vi "Teleop - Gyro Tracking (SubVI).vi"(0 "turretAngleDesiredInput":dbl=229.0, 1 "hoodAngleDesired In":dbl, 2 "shooterVelocityDesired In":dbl, 3 "shootNow In":bool, 4 "Constant Cluster In":T1 {"32. shooterHoodAngleRange" format="%_6f"; "31. turretAngleRange" format="%_6f"; "30. shooterVelocityLowerLimit" format="%_6f"; "29. shooterVelocityUpperLimit" format="%_6f"; "28. Robot Track Width (inches)" format="%_6f"; "27. Shooter Spin Up Speed (RPM)" format="%_6f"; "26. Climb Down Speed %" format="%_6f"; "25. Climb Up Speed %" format="%_6f"; "24. wallShooterVelocity" format="%_6f"; "23. Intake Spit Speed %" format="%_6f"; "22. Intake Suck Speed %" format="%_6f"; "21. CP Wheel Diameter" format="%_6f"; "20. Clockwise CP Fudge" format="%_6f"; "19. CouterClockwise CP Fudge" format="%_6f"; "18. Inches per Sector" format="%_6f"; "17. Ticks/Rotation Neo 550" format="%_6f"; "16. Control Panel Wheel Diameter" format="%_6f"; "15. Center-Center Sector Distance" format="%_6f"; "14. Inches / Tick Drivetrain" format="%_6f"; "13. Auton I Output Limit Drive Straight Gain" format="%_6f"; "12. Auton Deriv Drive Straight Gain" format="%_6f"; "11. Auton Int Drive Straight Gain" format="%_6f"; "10. Auton Prop Drive Straight Gain" format="%_6f"; "9. Auton I Output Limit Turn Gain" format="%_6f"; "8. Auton Deriv Turn Gain" format="%_6f"; "7. Auton Int Turn Gain" format="%_6f"; "1. Auton Prop Drive Gain" format="%_6f"; "2. Auton Int Drive Gain" format="%_6f"; "3. Auton Deriv Drive Gain" format="%_6f"; "4. I Output Drive  Limit" format="%_6f"; "5. Auto Drive Cheat (%)" format="%_6f"; "6. Auton Prop Turn Gain" format="%_6f"}, 5 "sensors In":T2) -> (15 "hoodAngleDesired Out":dbl, 16 "turretAngleDesiredOutput":dbl, 17 "shootNow Output":bool, 18 "Constant Cluster Out":T1 {"32. shooterHoodAngleRange" format="%_6f"; "31. turretAngleRange" format="%_6f"; "30. shooterVelocityLowerLimit" format="%_6f"; "29. shooterVelocityUpperLimit" format="%_6f"; "28. Robot Track Width (inches)" format="%_6f"; "27. Shooter Spin Up Speed (RPM)" format="%_6f"; "26. Climb Down Speed %" format="%_6f"; "25. Climb Up Speed %" format="%_6f"; "24. wallShooterVelocity" format="%_6f"; "23. Intake Spit Speed %" format="%_6f"; "22. Intake Suck Speed %" format="%_6f"; "21. CP Wheel Diameter" format="%_6f"; "20. Clockwise CP Fudge" format="%_6f"; "19. CouterClockwise CP Fudge" format="%_6f"; "18. Inches per Sector" format="%_6f"; "17. Ticks/Rotation Neo 550" format="%_6f"; "16. Control Panel Wheel Diameter" format="%_6f"; "15. Center-Center Sector Distance" format="%_6f"; "14. Inches / Tick Drivetrain" format="%_6f"; "13. Auton I Output Limit Drive Straight Gain" format="%_6f"; "12. Auton Deriv Drive Straight Gain" format="%_6f"; "11. Auton Int Drive Straight Gain" format="%_6f"; "10. Auton Prop Drive Straight Gain" format="%_6f"; "9. Auton I Output Limit Turn Gain" format="%_6f"; "8. Auton Deriv Turn Gain" format="%_6f"; "7. Auton Int Turn Gain" format="%_6f"; "1. Auton Prop Drive Gain" format="%_6f"; "2. Auton Int Drive Gain" format="%_6f"; "3. Auton Deriv Drive Gain" format="%_6f"; "4. I Output Drive  Limit" format="%_6f"; "5. Auto Drive Cheat (%)" format="%_6f"; "6. Auton Prop Turn Gain" format="%_6f"}, 19 "sensors Out":T2)   [LabVIEW 2019]
uses:
  Autonomous/TypeDefs/Sensor TypeDef.ctl
  Disabled/Constant VI_s/Disabled - Constant Cluster Typedef.ctl
panel:
  out "robotAngle":dbl
  out "angleToGoal":dbl
  in  "Goal X (in)":dbl=229.0
  in  "Goal Y (in)":dbl=629.25
  # "Input"
  # "Process"
  # "Output"
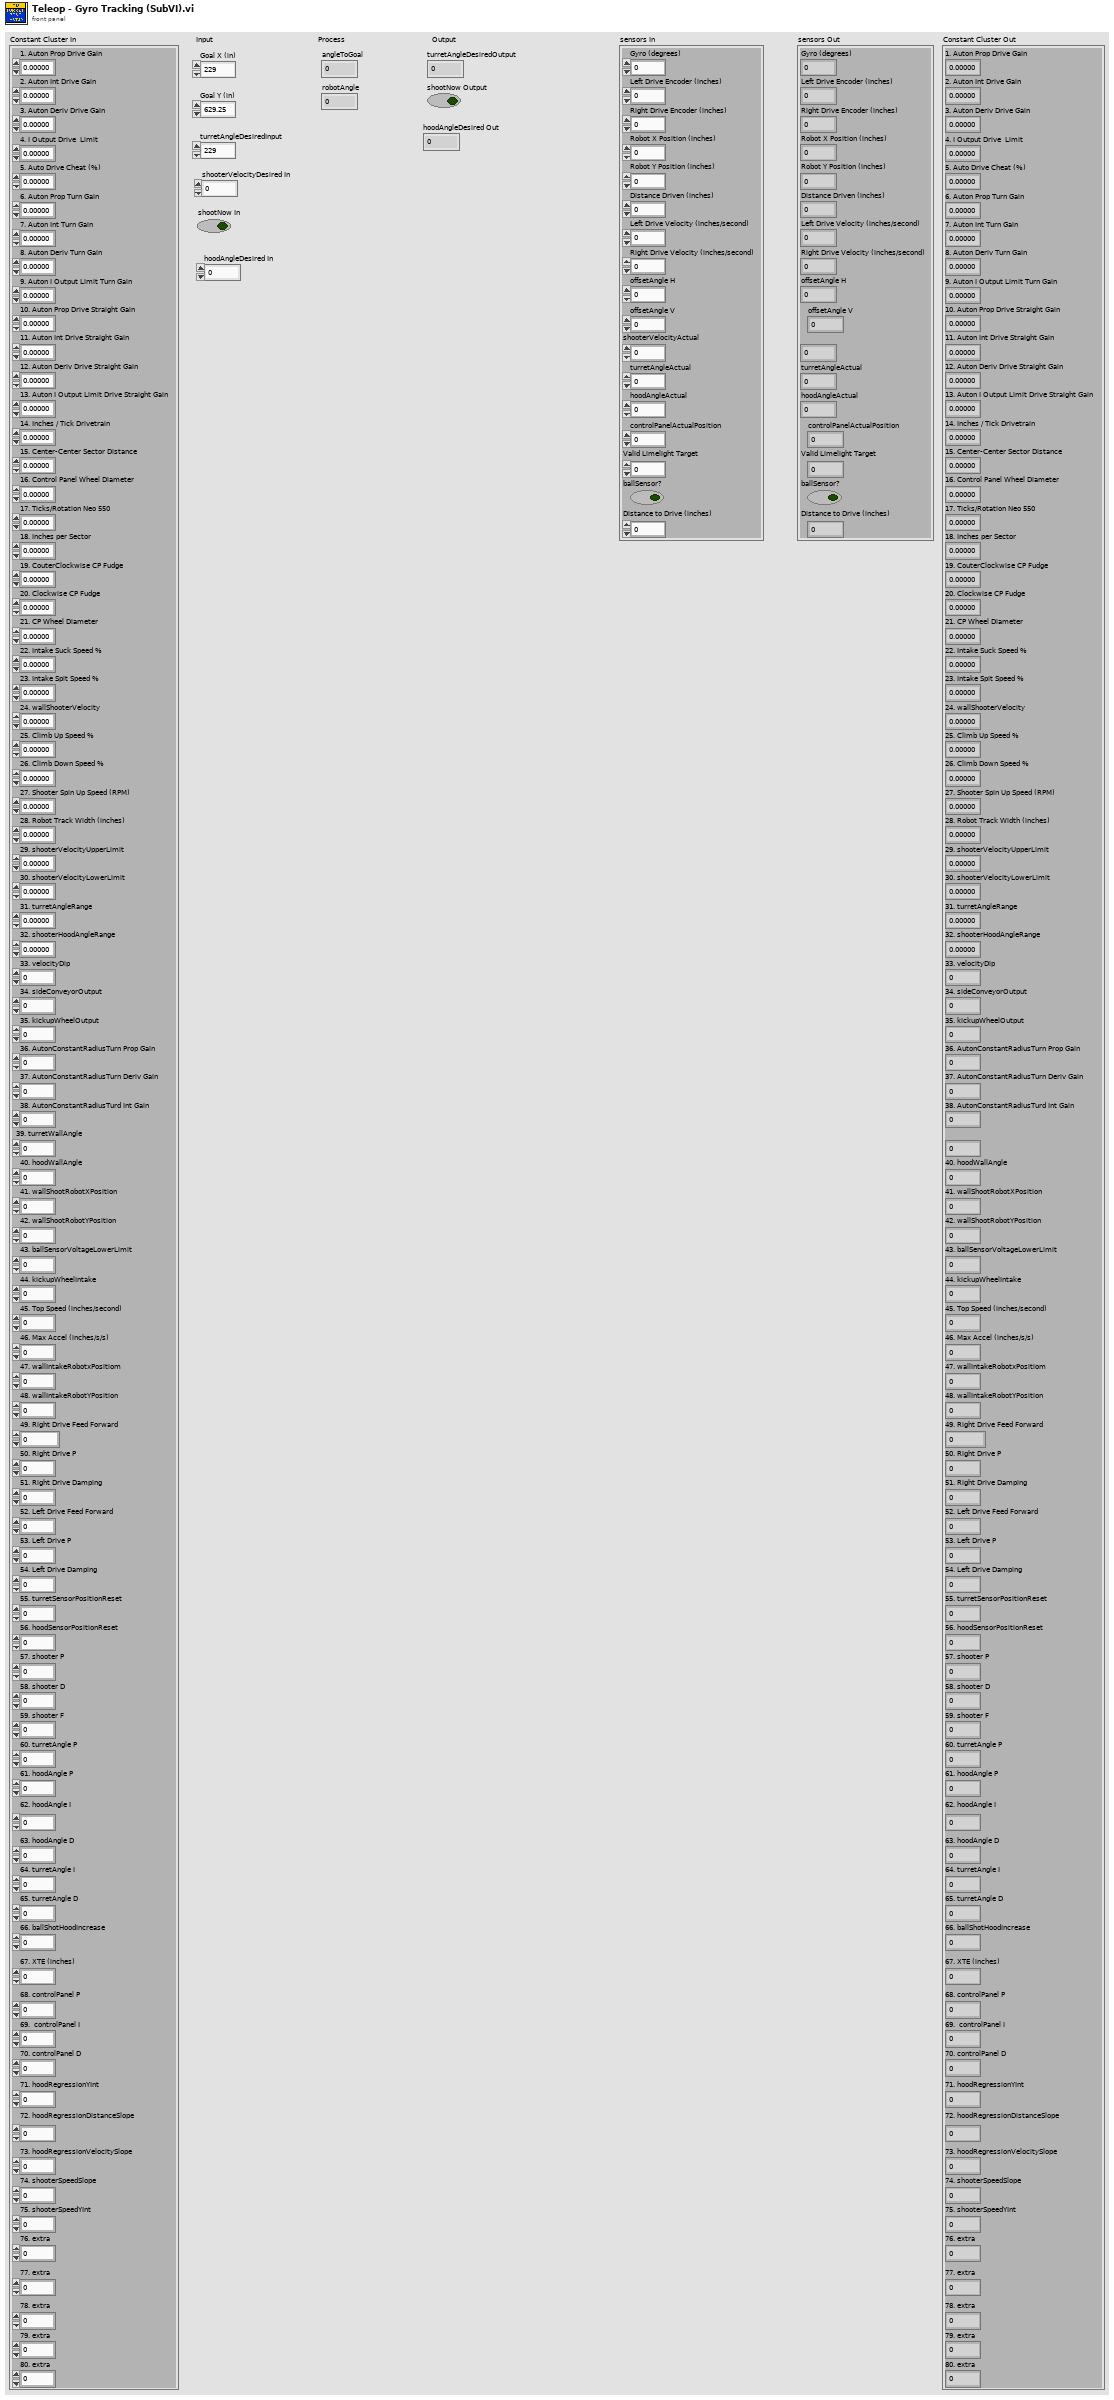
[diagram p1: front panel]
types:
  T1 = typedef "Disabled - Constant Cluster Typedef.ctl" = cluster{"1. Auton Prop Drive Gain":dbl, "2. Auton Int Drive Gain":dbl, "3. Auton Deriv Drive Gain":dbl, "4. I Output Drive  Limit":dbl, "5. Auto Drive Cheat (%)":dbl, "6. Auton Prop Turn Gain":dbl, "7. Auton Int Turn Gain":dbl, "8. Auton Deriv Turn Gain":dbl, "9. Auton I Output Limit Turn Gain":dbl, "10. Auton Prop Drive Straight Gain":dbl, "11. Auton Int Drive Straight Gain":dbl, "12. Auton Deriv Drive Straight Gain":dbl, "13. Auton I Output Limit Drive Straight Gain":dbl, "14. Inches / Tick Drivetrain":dbl, "15. Center-Center Sector Distance":dbl, "16. Control Panel Wheel Diameter":dbl, "17. Ticks/Rotation Neo 550":dbl, "18. Inches per Sector":dbl, "19. CouterClockwise CP Fudge":dbl, "20. Clockwise CP Fudge":dbl, "21. CP Wheel Diameter":dbl, "22. Intake Suck Speed %":dbl, "23. Intake Spit Speed %":dbl, "24. wallShooterVelocity":dbl, "25. Climb Up Speed %":dbl, "26. Climb Down Speed %":dbl, "27. Shooter Spin Up Speed (RPM)":dbl, "28. Robot Track Width (inches)":dbl, "29. shooterVelocityUpperLimit":dbl, "30. shooterVelocityLowerLimit":dbl, "31. turretAngleRange":dbl, "32. shooterHoodAngleRange":dbl, "33. velocityDip":dbl, "34. sideConveyorOutput":dbl, "35. kickupWheelOutput":dbl, "36. AutonConstantRadiusTurn Prop Gain":dbl, "37. AutonConstantRadiusTurn Deriv Gain":dbl, "38. AutonConstantRadiusTurd Int Gain":dbl, "39. turretWallAngle":dbl, "40. hoodWallAngle":dbl, "41. wallShootRobotXPosition":dbl, "42. wallShootRobotYPosition":dbl, "43. ballSensorVoltageLowerLimit":dbl, "44. kickupWheelIntake":dbl, "45. Top Speed (inches/second)":dbl, "46. Max Accel (inches/s/s)":dbl, "47. wallIntakeRobotxPositiom":dbl, "48. wallIntakeRobotYPosition":dbl, "49. Right Drive Feed Forward":dbl, "50. Right Drive P":dbl, "51. Right Drive Damping":dbl, "52. Left Drive Feed Forward":dbl, "53. Left Drive P":dbl, "54. Left Drive Damping":dbl, "55. turretSensorPositionReset":dbl, "56. hoodSensorPositionReset":dbl, "57. shooter P":dbl, "58. shooter D":dbl, "59. shooter F":dbl, "60. turretAngle P":dbl, "61. hoodAngle P":dbl, "62. hoodAngle I":dbl, "63. hoodAngle D":dbl, "64. turretAngle I":dbl, "65. turretAngle D":dbl, "66. ballShotHoodIncrease":dbl, "67. XTE (inches)":dbl, "68. controlPanel P":dbl, "69.  controlPanel I":dbl, "70. controlPanel D":dbl, "71. hoodRegressionYInt":dbl, "72. hoodRegressionDistanceSlope":dbl, "73. hoodRegressionVelocitySlope":dbl, "74. shooterSpeedSlope":dbl, "75. shooterSpeedYInt":dbl, "76. extra":dbl, "77. extra":dbl, "78. extra":dbl, "79. extra":dbl, "80. extra":dbl}
  T2 = typedef "Sensor TypeDef.ctl" = cluster{"Gyro (degrees)":dbl, "Left Drive Encoder (inches)":dbl, "Right Drive Encoder (inches)":dbl, "Robot X Position (inches)":dbl, "Robot Y Position (inches)":dbl, "Distance Driven (inches)":dbl, "Left Drive Velocity (inches/second)":dbl, "Right Drive Velocity (inches/second)":dbl, "offsetAngle H":dbl, "offsetAngle V":dbl, "shooterVelocityActual":dbl, "turretAngleActual":dbl, "hoodAngleActual":dbl, "controlPanelActualPosition":dbl, "Valid Limelight Target":dbl, "ballSensor?":bool, "Distance to Drive (inches)":dbl}
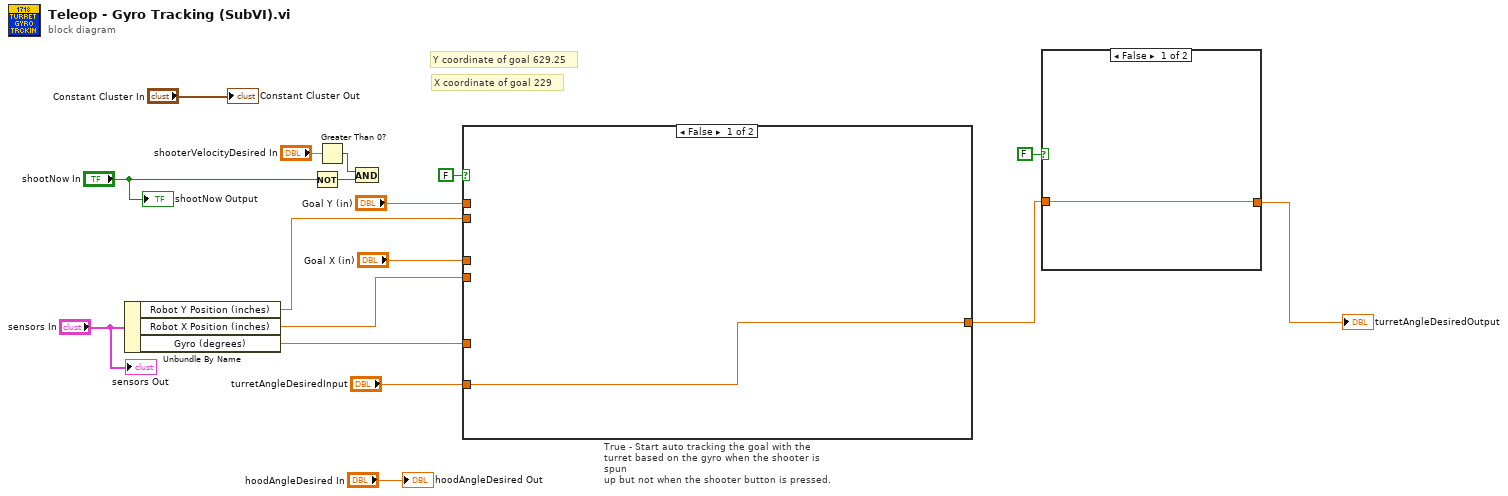
[diagram p0: block diagram]
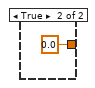
[diagram p2: hidden frame]
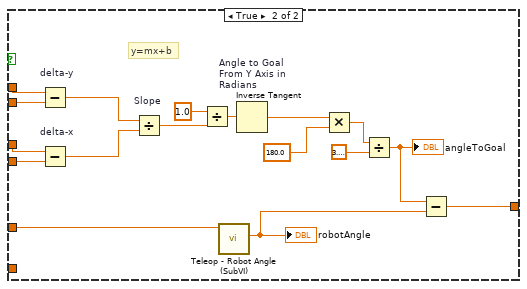
[diagram p3: hidden frame]
diagram:
  # "X coordinate of goal 229"
  # "Y coordinate of goal 629.25"
  n1 = Unbundle By Name("sensors In") -> ("Robot Y Position (inches)"=w10:dbl, "Robot X Position (inches)"=w12:dbl, "Gyro (degrees)"=w11:dbl)
  n2 = Not(x="shootNow In") -> (.not. x?=w16:bool)
  n3 = Greater Than 0?(x="shooterVelocityDesired In") -> (x > 0?=w17:bool)
  n4 = And(x=w17, y=w16) -> ()  [unwired: 1 out]
  n5 = case "True - Start auto tracking the goal with the turret based on the gyro when the shooter is spun\nup but not when the shooter button is pressed." shown="False" FALSE {
    tunnel: w11 -> [_ w21]
    tunnel: "Goal X (in)" -> [_ w35]
    tunnel: w12 -> [_ w34]
    tunnel: "Goal Y (in)" -> [_ w33]
    tunnel: w10 -> [_ w32]
    tunnel: [w18 w20] -> w3
    tunnel: "turretAngleDesiredInput" -> [w18 _]
    frame False {
    }
    frame True {
      # "y=mx+b"
      n6 = Subtract "delta-y"(x=w33, y=w32) -> (x-y=w30:dbl)
      n7 = Subtract "delta-x"(x=w35, y=w34) -> (x-y=w31:dbl)
      n8 = Divide "Slope"(x=w30, y=w31) -> (x/y=w28:dbl)
      n9 = Divide(x=1.0, y=w28) -> (x/y=w27:dbl)
      n10 = call "Teleop - Robot Angle (SubVI).vi"("yaw in"=w21) -> ("angle"=w19:dbl)  [unwired: 10 in]
      "robotAngle" <- w19
      n11 = Inverse Tangent "Angle to Goal\nFrom Y Axis in\nRadians"(1:w27) -> (0:w26:dbl)
      n12 = Multiply(x=w26, y=180.0) -> (x*y=w24:dbl)
      n13 = Divide(x=w24, y=3.141592653589793) -> (x/y=w22:dbl)
      "angleToGoal" <- w22
      n14 = Subtract(x=w22, y=w19) -> (x-y=w20:dbl)
    }
  }
  n15 = case shown="False" FALSE {
    tunnel: w3 -> [w36 _]
    tunnel: [w36 0.0 ("turretAngleDesiredInput")] -> w2
    frame False {
    }
    frame True {
    }
  }
  "turretAngleDesiredOutput" <- w2
  "sensors Out" <- "sensors In"
  "shootNow Output" <- "shootNow In"
  "hoodAngleDesired Out" <- "hoodAngleDesired In"
  "Constant Cluster Out" <- "Constant Cluster In"
